vi "Create Multipart Content.vi"(5 "HttpContent_Multipart in":refnum<class "HttpContent_Multipart.lvclass">, 6 "boundary":string, 8 "error in (no error)":errorcluster, 11 "multipart type":T1="multipart/mixed") -> (0 "error out":errorcluster, 3 "HttpContent_Multipart out":refnum<class "HttpContent_Multipart.lvclass">)   [LabVIEW 2018, in "LabVIEWHTTPClient_NET.lvlib" / "HttpContent_Multipart.lvclass"]
uses:
  HttpContent_Multipart.lvclass
  C:/Viviota/Projects/R&D/LabVIEW_HTTP_REST_NET/HttpContent/HttpContent.lvclass
  Types/multipart_types_combo.ctl
  System.Net.Http
  HttpContent/HttpContent.lvclass
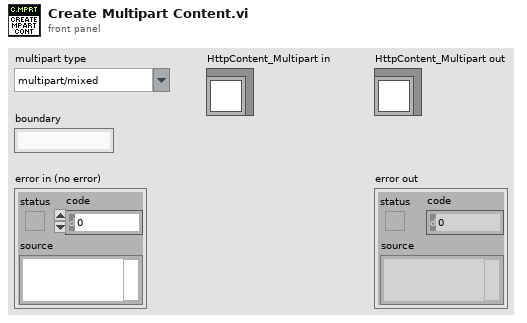
[diagram p1: front panel]
types:
  T1 = typedef "LabVIEWHTTPClient_NET.lvlib/HttpContent_Multipart.lvclass/multipart_types_combo.ctl" = string
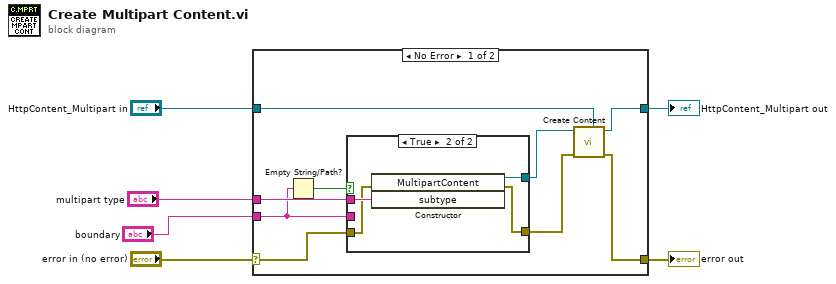
[diagram p0: block diagram]
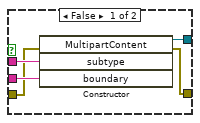
[diagram p2: hidden frame]
diagram:
  n1 = case shown="No Error" "error in (no error)" {
    selector: "error in (no error)" -> [w12 w26]
    tunnel: [w8 w26] -> w5
    tunnel: [w10 w25] -> w3
    tunnel: "HttpContent_Multipart in" -> [w11 w25]
    tunnel: "multipart type" -> [w15 _]
    tunnel: "boundary" -> [w14 _]
    frame No Error {
      n2 = Empty String/Path?(string/path=w14) -> (empty?=w13:bool)
      n3 = case shown="True" w13 {
        tunnel: w15 -> [w20 w24]
        tunnel: w14 -> [w19 _]
        tunnel: [w17 w23] -> w7
        tunnel: w12 -> [w18 w22]
        tunnel: [w16 w21] -> w9
        frame False {
          n4 = constructor class="MultipartContent"(error in=w18, "subtype"=w20, "boundary"=w19) -> (reference out=w17:refnum<k24>, error out=w16:errorcluster)  [unwired: 2 in, 3 out]
        }
        frame True {
          n5 = constructor class="MultipartContent"(error in=w22, "subtype"=w24) -> (reference out=w23:refnum<k24>, error out=w21:errorcluster)  [unwired: 2 in, 2 out]
        }
      }
      n6 = call "Create Content.vi"("HttpContent in"=w11, "error in (no error)"=w9, "NET_HttpContent"=w7) -> ("error out"=w8:errorcluster, "HttpContent out"=w10:refnum<class "HttpContent_Multipart.lvclass">)  [unwired: 7 in]
    }
    frame Error {
    }
  }
  "error out" <- w5
  "HttpContent_Multipart out" <- w3
